vi "Global Data!!!.vi"() -> ()   [LabVIEW 2014]
panel:
  in  "accelInfo":T1
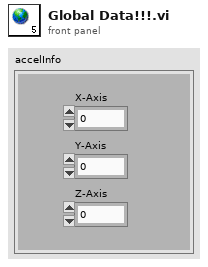
[diagram p1: front panel]
types:
  T1 = cluster{"X-Axis":dbl, "Y-Axis":dbl, "Z-Axis":dbl}
diagram:
